vi "Stop Controller.vi"(8 "error in (no error)":errorcluster, 10 "Close UI?":bool, 11 "TestStand Controller Queue":refnum<class "Message Enqueuer.lvclass">) -> (0 "error out":errorcluster)   [LabVIEW 2016, in "Controller API.lvlib" / "Controller API.lvclass"]
uses:
  Controller API.lvclass
  <vilib>/ActorFramework/Message Enqueuer/Message Enqueuer.lvclass
  <vilib>/ActorFramework/Message Enqueuer/Message Enqueuer.lvclass/Message Enqueuer.ctl
  <vilib>/ActorFramework/Message Enqueuer/Enqueue.vi
  <vilib>/ActorFramework/Stop Msg/Stop Msg.lvclass
  C:/Program Files (x86)/National Instruments/LabVIEW 2016/vi.lib/ActorFramework/Message/Message.lvclass
  <vilib>/ActorFramework/Message Priority Queue/Priority Enqueue.vi
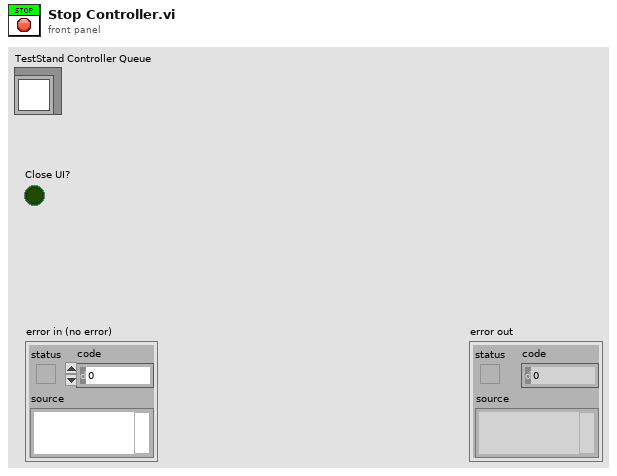
[diagram p1: front panel]
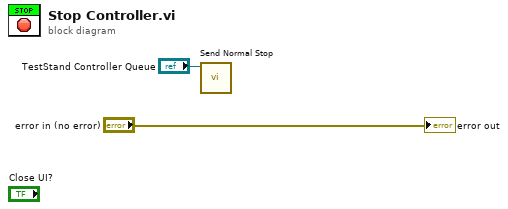
[diagram p0: block diagram]
diagram:
  n1 = call <vilib>:"Send Normal Stop.vi"("Message Enqueuer"="TestStand Controller Queue") -> ()  [unwired: 10 in, 1 out]
  "error out" <- "error in (no error)"
